vi "LEDSocketKit.vi"() -> ()   [LabVIEW 2024]
uses:
  Driver/Public/Digital Direction.ctl
  Driver/CTIPicoVISA.lvlib
panel:
  out "Boolean":bool
  out "Identity":T1
  in  "GroveConnector":enum16{"D16", "D18", "D20"}(ring)
  in  "stop":bool
  in  "VISA resource name in":refnum<visa-resource-name>
  out "error out":errorcluster
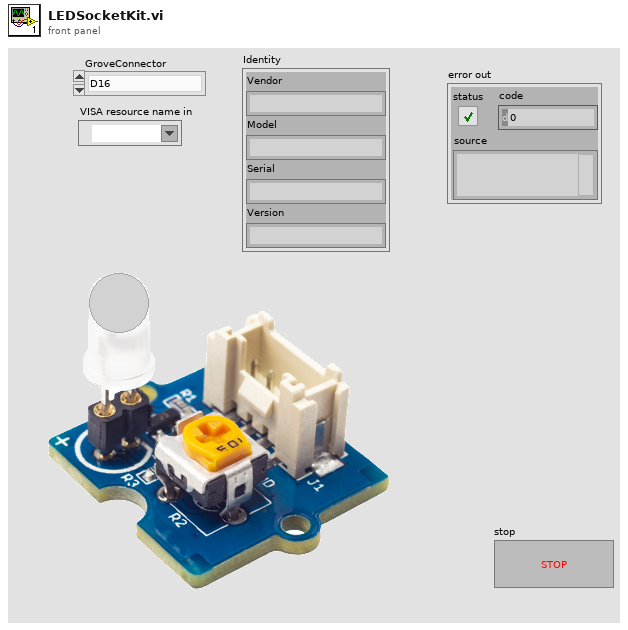
[diagram p1: front panel]
types:
  T1 = cluster{"Vendor":string, "Model":string, "Serial":string, "Version":string}
  T2 = typedef "CTIPicoVISA.lvlib/Digital Direction.ctl" = enum16{"In", "Out"}
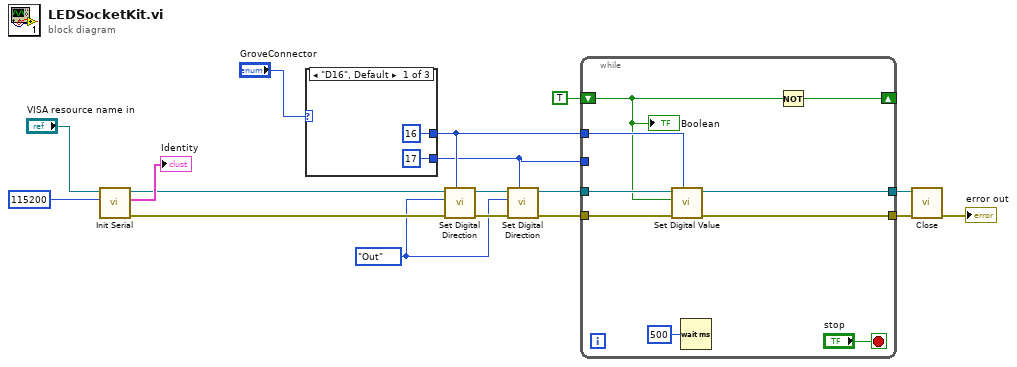
[diagram p0: block diagram]
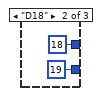
[diagram p2: hidden frame]
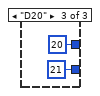
[diagram p3: hidden frame]
diagram:
  w9 = Digital_Direction."Out" ("Direction")
  n1 = call "Init Serial.vi"("Baud (115200)"=u32 115200, "VISA resource name in"="VISA resource name in") -> ("error out"=w11:errorcluster, "Identity"=→"Identity":T1, "VISA resource name Out"=w13:refnum<visa-resource-name>)  [unwired: 7 in]
  n2 = case shown="\"D16\", Default" "GroveConnector" {
    tunnel: [16 ("GPIO") 18 ("GPIO") 20 ("GPIO")] -> w12
    tunnel: [17 ("GPIO") 19 ("GPIO") 21 ("GPIO")] -> w7
    frame "D16", Default {
    }
    frame "D18" {
    }
    frame "D20" {
    }
  }
  n3 = call "Set Digital Direction.vi"("GPIO"=w12, "error in (no error)"=w11, "Direction"=w9, "VISA resource name in"=w13) -> ("error out"=w10:errorcluster, "VISA resource name"=w8:refnum<visa-resource-name>)  [unwired: 6 in]
  n4 = call "Set Digital Direction.vi"("GPIO"=w7, "error in (no error)"=w10, "Direction"=w9, "VISA resource name in"=w8) -> ("error out"=w5:errorcluster, "VISA resource name"=w6:refnum<visa-resource-name>)  [unwired: 6 in]
  n5 = while {
    tunnel: w5 -> [w29]
    tunnel: w6 -> [w30]
    tunnel: [w25] -> w4
    tunnel: [w24] -> w3
    tunnel: w12 -> [w28]
    tunnel: w7 -> [_]
    shift-right: [w26] -> _
    shift-left: TRUE -> [w27]
    stop <- "stop" stop-if-true
    n6 = call "Set Digital Value.vi"("GPIO"=w28, "error in (no error)"=w29, "Value"=w27, "VISA resource name in"=w30) -> ("error out"=w24:errorcluster, "VISA resource name"=w25:refnum<visa-resource-name>)  [unwired: 6 in]
    n7 = Wait (ms)(milliseconds to wait=u32 500) -> ()  [unwired: 1 out]
    n8 = Not(x=w27) -> (.not. x?=w26:bool)
    "Boolean" <- w27
  }
  n9 = call "Close.vi"("error in (no error)"=w3, "VISA resource name in"=w4) -> ("error out"=→"error out":errorcluster)  [unwired: 9 in]
